vi "MeasurementServer_Start.vi"(7 "error in (no error)":errorcluster, 8 "Server Key File (.key)":path, 9 "Server Certificate File (.crt)":path, 10 "Server Address":string) -> (0 "error out":errorcluster, 2 "Event Registration Refnum":refnum<event-registration>, 3 "Server Information":T2)   [LabVIEW 2019, in "labview-grpc-measurement-server.lvlib"]
uses:
  labview-grpc-measurement-server.lvlib
  MeasurementServer_InvokeEventData.ctl
  MeasurementServer_gRPCid.ctl
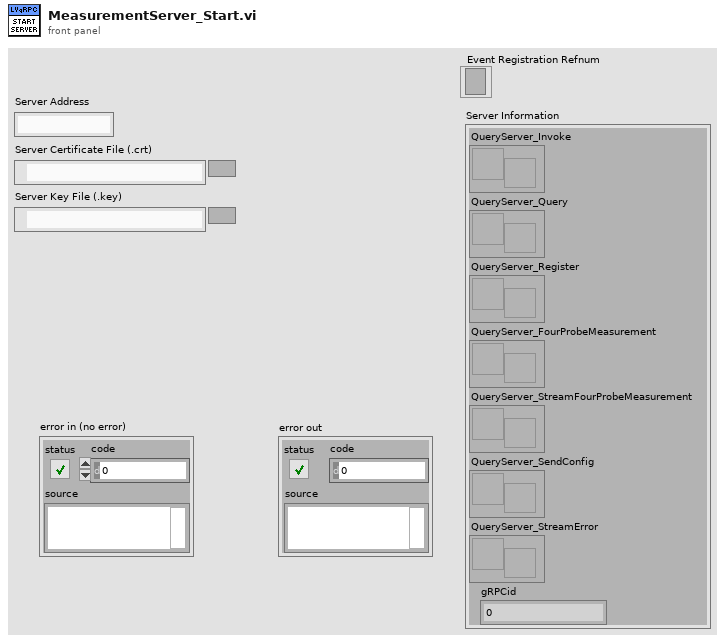
[diagram p1: front panel]
types:
  T1 = typedef "labview-grpc-measurement-server.lvlib/MeasurementServer_gRPCid.ctl" = u64
  T2 = cluster{"QueryServer_Invoke":refnum<user-event>, "QueryServer_Query":refnum<user-event>, "QueryServer_Register":refnum<user-event>, "QueryServer_FourProbeMeasurement":refnum<user-event>, "QueryServer_StreamFourProbeMeasurement":refnum<user-event>, "QueryServer_SendConfig":refnum<user-event>, "QueryServer_StreamError":refnum<user-event>, "gRPCid":T1}
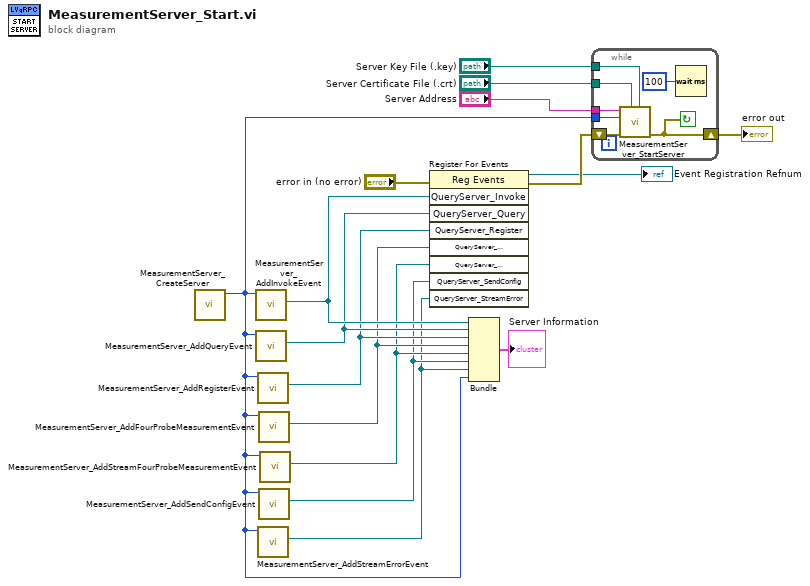
[diagram p0: block diagram]
diagram:
  n1 = call "MeasurementServer_CreateServer.vi"() -> ("gRPCid"=w4:T1)  [unwired: 11 in]
  n2 = call "MeasurementServer_AddInvokeEvent.vi"("gRPCid in"=w4) -> ("QueryServer_Invoke"=w11:refnum<user-event>)  [unwired: 9 in, 1 out]
  n3 = call "MeasurementServer_AddQueryEvent.vi"("gRPCid in"=w4) -> ("QueryServer_Query"=w10:refnum<user-event>)  [unwired: 9 in, 1 out]
  n4 = call "MeasurementServer_AddRegisterEvent.vi"("gRPCid in"=w4) -> ("QueryServer_Register"=w9:refnum<user-event>)  [unwired: 9 in, 1 out]
  n5 = call "MeasurementServer_AddStreamErrorEvent.vi"("gRPCid in"=w4) -> ("QueryServer_StreamError"=w3:refnum<user-event>)  [unwired: 9 in, 1 out]
  n6 = call "MeasurementServer_AddFourProbeMeasurementEvent.vi"("gRPCid in"=w4) -> ("QueryServer_FourProbeMeasurement"=w8:refnum<user-event>)  [unwired: 9 in, 1 out]
  n7 = call "MeasurementServer_AddSendConfigEvent.vi"("gRPCid in"=w4) -> ("QueryServer_SendConfig"=w5:refnum<user-event>)  [unwired: 9 in, 1 out]
  n8 = call "MeasurementServer_AddStreamFourProbeMeasurementEvent.vi"("gRPCid in"=w4) -> ("QueryServer_StreamFourProbeMeasurement"=w7:refnum<user-event>)  [unwired: 9 in, 1 out]
  n9 = register-events(error in="error in (no error)", w11, w10, w9, w8, w7, w5, w3) -> (reference out=→"Event Registration Refnum":refnum<event-registration>, error out=w12:errorcluster)  [unwired: 1 in]
  n10 = Bundle("QueryServer_Invoke"=w11, "QueryServer_Query"=w10, "QueryServer_Register"=w9, "QueryServer_FourProbeMeasurement"=w8, "QueryServer_StreamFourProbeMeasurement"=w7, "QueryServer_SendConfig"=w5, "QueryServer_StreamError"=w3, "gRPCid"=w4) -> (→"Server Information":T2)  [unwired: 1 in]
  n11 = while {
    tunnel: "Server Address" -> [w23]
    tunnel: "Server Certificate File (.crt)" -> [w22]
    tunnel: "Server Key File (.key)" -> [w21]
    tunnel: w4 -> [w19]
    shift-right: [w18] -> w6
    shift-left: w12 -> [w20]
    stop <- w18 continue-if-true
    n12 = call "MeasurementServer_StartServer.vi"("Server Key File (.key)"=w21, "Server Certificate File (.crt)"=w22, "error in (no error)"=w20, "gRPCid"=w19, "Server Address"=w23) -> ("error out"=w18:errorcluster)  [unwired: 6 in]
    n13 = Wait (ms)(milliseconds to wait=u32 100) -> ()  [unwired: 1 out]
  }
  "error out" <- w6
